vi "Frameproperties_raw.vi"(11 "array":dbl[][](array[numeric])) -> (3 "Frame properties":cluster{cluster{dbl, dbl}, cluster{dbl, dbl}})   [LabVIEW 2017]
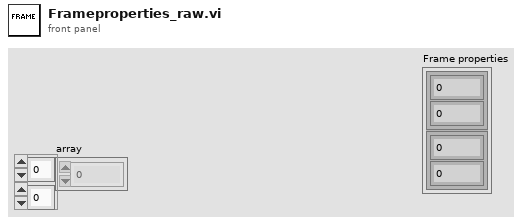
[diagram p1: front panel]
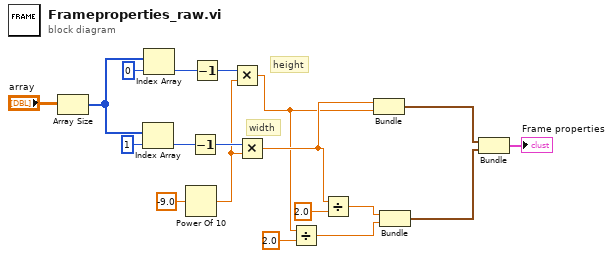
[diagram p0: block diagram]
diagram:
  # "width"
  # "height"
  n1 = Array Size(array="array") -> (size(s)=w18:i32[])
  n2 = Index Array(array=w18, index=1) -> (element=w14:i32)
  n3 = Index Array(array=w18, index=0) -> (element=w15:i32)
  n4 = Power Of 10(x=-9.0) -> (10^x=w11:dbl)
  n5 = Decrement(x=w14) -> (x-1=w12:i32)
  n6 = Decrement(x=w15) -> (x-1=w13:i32)
  n7 = Multiply(x=w13, y=w11) -> (x*y=w6:dbl)
  n8 = Multiply(x=w12, y=w11) -> (x*y=w9:dbl)
  n9 = Divide(x=w6, y=2.0) -> (x/y=w4:dbl)
  n10 = Divide(x=w9, y=2.0) -> (x/y=w5:dbl)
  n11 = Bundle(w9, w6) -> (w3:cluster{dbl, dbl})  [unwired: 1 in]
  n12 = Bundle(w5, w4) -> (w2:cluster{dbl, dbl})  [unwired: 1 in]
  n13 = Bundle(w3, w2) -> (→"Frame properties":cluster{cluster{dbl, dbl}, cluster{dbl, dbl}})  [unwired: 1 in]
